vi "datatapyes.vi"() -> ()   [LabVIEW 2020]
panel:
  out "StrInd":string
  in  "Strctrl":string
  out "BoolInd":bool
  out "int Ind":u8
  in  "int ctrl":u8
  in  "Boolctrl":bool
  out "NumInd":dbl
  in  "Numctrl":dbl
  # "Data types"
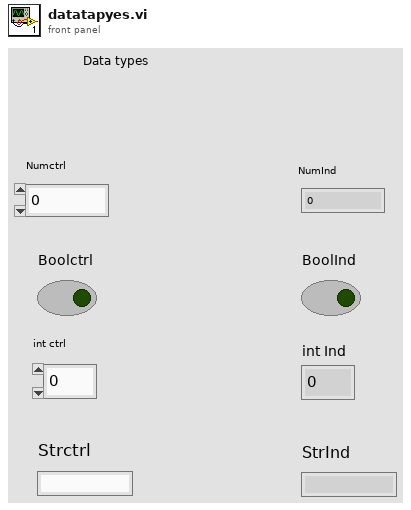
[diagram p1: front panel]
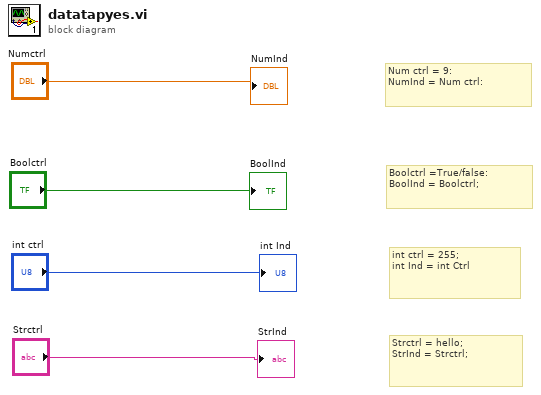
[diagram p0: block diagram]
diagram:
  # "Strctrl = hello;\nStrInd = Strctrl;"
  # "int ctrl = 255;\nint Ind = int Ctrl"
  # "Boolctrl =True/false:\nBoolInd = Boolctrl;"
  # "Num ctrl = 9:\nNumInd = Num ctrl:"
  "NumInd" <- "Numctrl"
  "int Ind" <- "int ctrl"
  "BoolInd" <- "Boolctrl"
  "StrInd" <- "Strctrl"
